vi "GetNUmberOfCleaners.vi"(0 "object in":refnum<class "Value.lvclass">, 11 "Error In":errorcluster) -> (4 "object out":refnum<class "Value.lvclass">, 15 "Error Out":errorcluster)   [LabVIEW 2018, in "Value.lvclass"]
uses:
  Value.lvclass
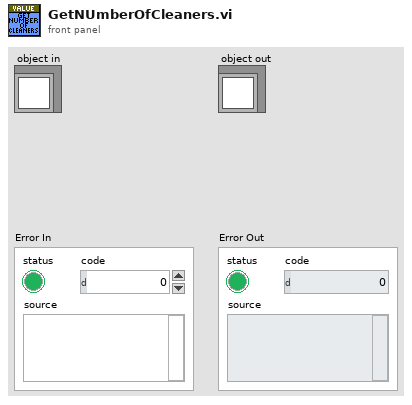
[diagram p1: front panel]
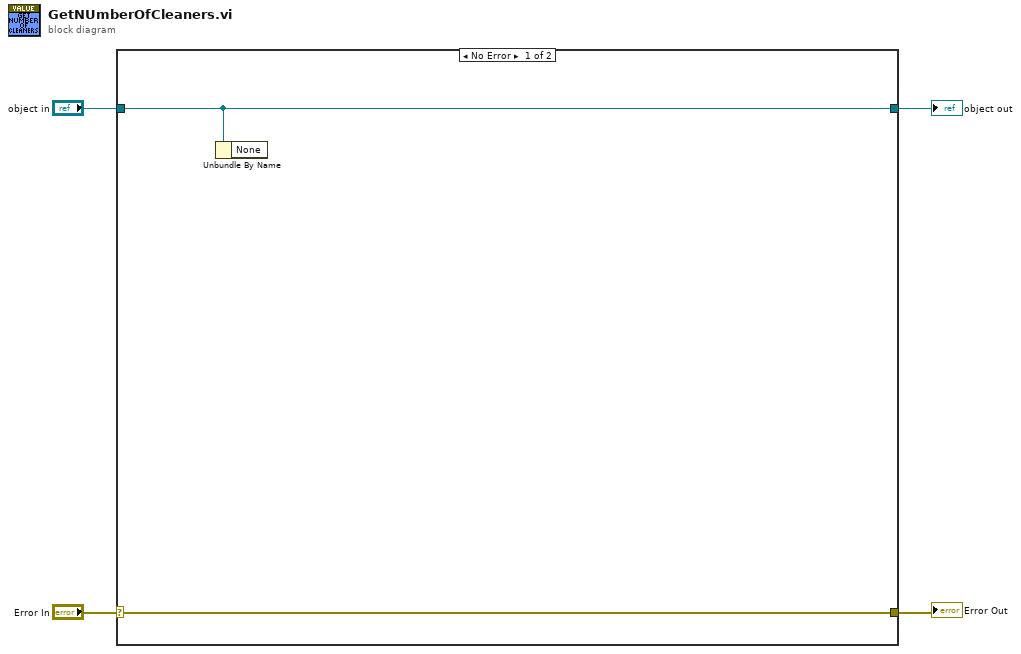
[diagram p0: block diagram]
diagram:
  n1 = case shown="No Error" "Error In" {
    selector: "Error In" -> [w6 w8]
    tunnel: [w6 w8] -> w3
    tunnel: [w5 w7] -> w1
    tunnel: "object in" -> [w5 w7]
    frame No Error {
      n2 = Unbundle By Name(w5) -> ()  [unwired: 1 out]
    }
    frame Error {
    }
  }
  "Error Out" <- w3
  "object out" <- w1
